vi "Open.vi"(8 "error in (no error)":errorcluster) -> (0 "error out":errorcluster)   [LabVIEW 2015]
uses:
  <vilib>/Rock Robotics/SystemInterfaces/i2clib/i2c_bus.ctl
  <vilib>/Rock Robotics/SystemInterfaces/DIO/FPGA_DIOChannel.ctl
  <vilib>/Rock Robotics/SystemInterfaces/AI/FPGA_AIChannel.ctl
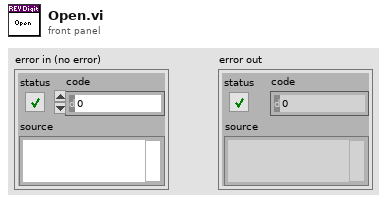
[diagram p1: front panel]
types:
  T1 = typedef "FPGA_AIChannel.ctl" = enum8{"AI 0", "AI 1", "AI 2", "AI 3", "AI MXP 0", "AI MXP 1", "AI MXP 2", "AI MXP 3", "Invalid"}
  T2 = typedef "FPGA_DIOChannel.ctl" = enum8{"DIO 0", "DIO 1", "DIO 2", "DIO 3", "DIO 4", "DIO 5", "DIO 6", "DIO 7", "DIO 8", "DIO 9", "DIO MXP 0", "DIO MXP 1", "DIO MXP 2", "DIO MXP 3", "DIO MXP 4", "DIO MXP 5", "DIO MXP 6", "DIO MXP 7", "DIO MXP 8", "DIO MXP 9", "DIO MXP 10", "DIO MXP 11", "DIO MXP 12", "DIO MXP 13", "DIO MXP 14", "DIO MXP 15", "Invalid"}
  T3 = typedef "i2c_bus.ctl" = enum16{"I2C On-Board", "I2C MXP", "Invalid"}
  T4 = typedef "WPI_I2CDevRef.ctl" = cluster{"DevStatus":errorcluster, "Device Address":u8, "Handle":i32, "I2C Bus":T3}
  T5 = typedef "WPI_DigitalInputDevRef.ctl" = cluster{"DevStatus":errorcluster, "DIO Channel":T2}
  T6 = typedef "WPI_AnalogChannelDevRef.ctl" = cluster{"DevStatus":errorcluster, "Analog Channel":T1}
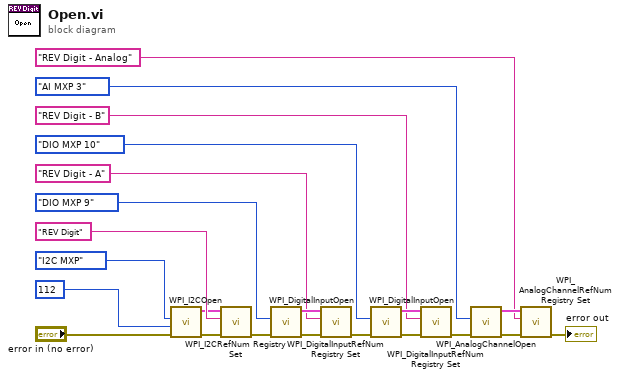
[diagram p0: block diagram]
diagram:
  n1 = call <vilib>:"WPI_I2COpen.vi"("error in"="error in (no error)", "Device Address"=u8 112, "I2C Bus"=i2c_bus."I2C MXP") -> ("error out"=w21:errorcluster, "I2CDevRef"=w20:T4)  [unwired: 7 in]
  n2 = call <vilib>:"WPI_I2CRefNum Registry Set.vi"("error in (no error)"=w21, "refnum name"="REV Digit", "I2CDevRef"=w20) -> ("error out"=w4:errorcluster)  [unwired: 7 in, 1 out]
  n3 = call <vilib>:"WPI_DigitalInputOpen.vi"("error in (no error)"=w4, "DIO Channel"=FPGA_DIOChannel."DIO MXP 9") -> ("error out"=w16:errorcluster, "DigitalInputDevRef"=w15:T5)  [unwired: 8 in]
  n4 = call <vilib>:"WPI_DigitalInputRefNum Registry Set.vi"("error in (no error)"=w16, "refnum name"="REV Digit - A", "DigitalInputDevRef"=w15) -> ("error out"=w3:errorcluster)  [unwired: 7 in, 1 out]
  n5 = call <vilib>:"WPI_DigitalInputOpen.vi"("error in (no error)"=w3, "DIO Channel"=FPGA_DIOChannel."DIO MXP 10") -> ("error out"=w14:errorcluster, "DigitalInputDevRef"=w13:T5)  [unwired: 8 in]
  n6 = call <vilib>:"WPI_DigitalInputRefNum Registry Set.vi"("error in (no error)"=w14, "refnum name"="REV Digit - B", "DigitalInputDevRef"=w13) -> ("error out"=w2:errorcluster)  [unwired: 7 in, 1 out]
  n7 = call <vilib>:"WPI_AnalogChannelOpen.vi"("error in (no error)"=w2, "Analog Channel"=FPGA_AIChannel."AI MXP 3") -> ("error out"=w8:errorcluster, "AIDeviceRef"=w7:T6)  [unwired: 8 in]
  n8 = call <vilib>:"WPI_AnalogChannelRefNum Registry Set.vi"("error in (no error)"=w8, "refnum name"="REV Digit - Analog", "AIDeviceRef"=w7) -> ("error out"=→"error out":errorcluster)  [unwired: 7 in, 1 out]
